vi "PPMS3.Remote Client.vi"(8 "error in (no error)":errorcluster, 9 "Data":variant, 10 "Command":T1, 11 "instrument.PPMS3 in":refnum<class "instrument.PPMS3.lvclass">) -> (0 "error out":errorcluster, 1 "Data out":variant, 2 "Command out":string, 3 "instrument.PPMS3 out":refnum<class "instrument.PPMS3.lvclass">)   [LabVIEW 2016, in "instrument.PPMS3.lvclass"]
uses:
  instrument.PPMS3.lvclass
  C:/Program Files (x86)/National Instruments/LabVIEW 2016/user.lib/LevyLab/Levylab Instruments/SMOs/Instrument/Instrument.lvclass
  Typedefs/PPMS3.Commands-enum.ctl
  <userlib>/LevyLab/Levylab Instruments/SMOs/Instrument/Instrument.lvclass
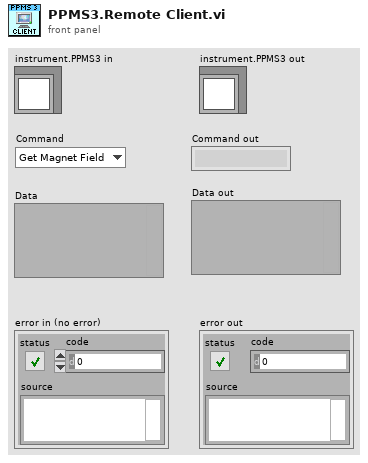
[diagram p1: front panel]
types:
  T1 = typedef "instrument.PPMS3.lvclass/PPMS3.Commands-enum.ctl" = enum16{"Get Magnet Field", "Get Helium Level", "Get Temperature", "Set Magnet Field", "Set Temperature", "getAll"}
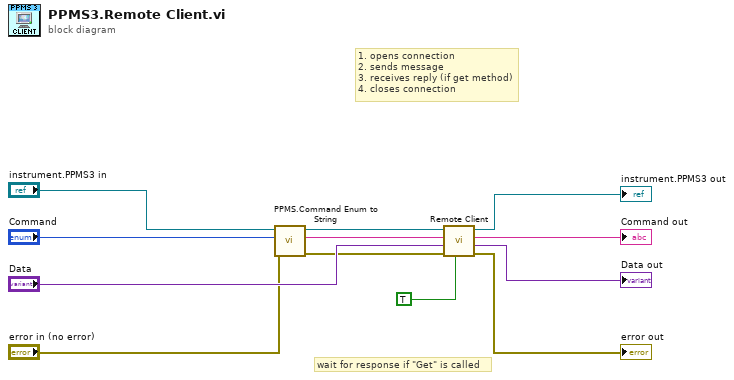
[diagram p0: block diagram]
diagram:
  # "1. opens connection\n2. sends message\n3. receives reply (if get method)\n4. closes connection"
  # "wait for response if \"Get\" is called"
  n1 = call "PPMS.Command Enum to String.vi"("error in (no error)"="error in (no error)", "Command"="Command", "instrument.PPMS in"="instrument.PPMS3 in") -> ("error out"=w3:errorcluster, "Command"=w5:string, "instrument.PPMS out"=w2:refnum<class "instrument.PPMS3.lvclass">)  [unwired: 5 in, 1 out]
  n2 = call <userlib>:"Remote Client.vi"("Wait for Response? [T]"=TRUE ("Wait for Response?"), "error in (no error)"=w3, "Data"="Data", "Command"=w5, "Instrument in"=w2) -> ("error out"=→"error out":errorcluster, "Data out"=→"Data out":variant, "Command out"=→"Command out":string, "Instrument out"=→"instrument.PPMS3 out":refnum<class "instrument.PPMS3.lvclass">)  [unwired: 3 in]
